vi "Teste Substrato Flexível 0.1_2025.vi"() -> ()   [LabVIEW 2019]
panel:
  in  "Zero":bool
  out "Posição":dbl
  out "T (s)":dbl format="%#_3g"
  out "F (hz)":dbl format="%#_3g"
  out "Tempo (s)":u32
  out "init":u32
  out "In LOOP":bool
  out "Close":bool
  out "Open":bool
  in  "Loop Stop":i32=50 min=1
  in  "Loop Stop":bool
  in  "stop":bool
  in  "Loop Infinito":bool
  out "Vel Cte":i32
  in  "Vel Loop":i32(slide)=20 min=10 max=200 step=5 scale=10.0..200.0
  in  "Jog":i32=10
  in  "Jog_s":string="10"
  in  "Desl_s":string="50"
  out "Contador":dbl format="%.2f"
  in  "Power Off":bool
  in  "Down":bool
  in  "Up":bool
  out "read buffer":string
  out "Direcção":bool
  out "error":errorcluster
  in  "Arduino":refnum<visa-resource-name>="COM3"
  # "Controle Mecanismo Teste de Substrato Flexível"
  # "LOEM"
  # "Velocidade de Deslocamento"
  # "Contador de Ciclos"
  # "Parar em ciclo"
  # "CONTROLE MANUAL"
  # "Pg Down"
  # "Pg Up"
  # "Steps"
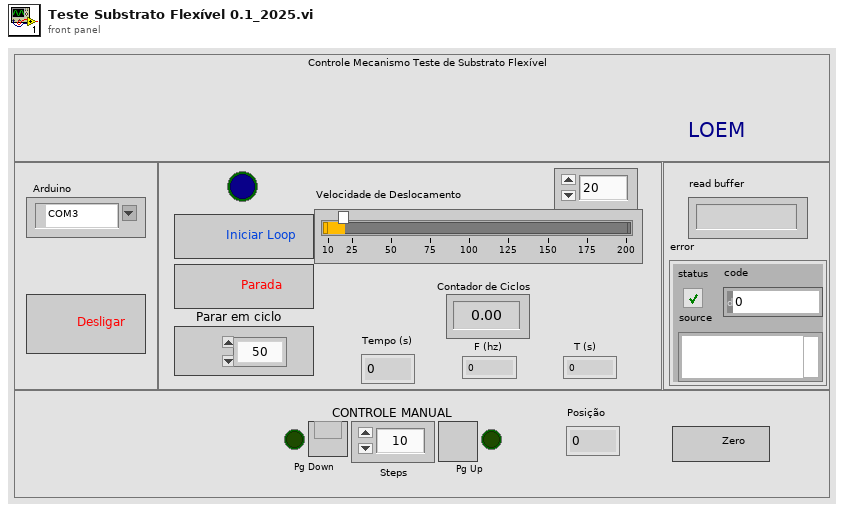
[diagram p1: front panel]
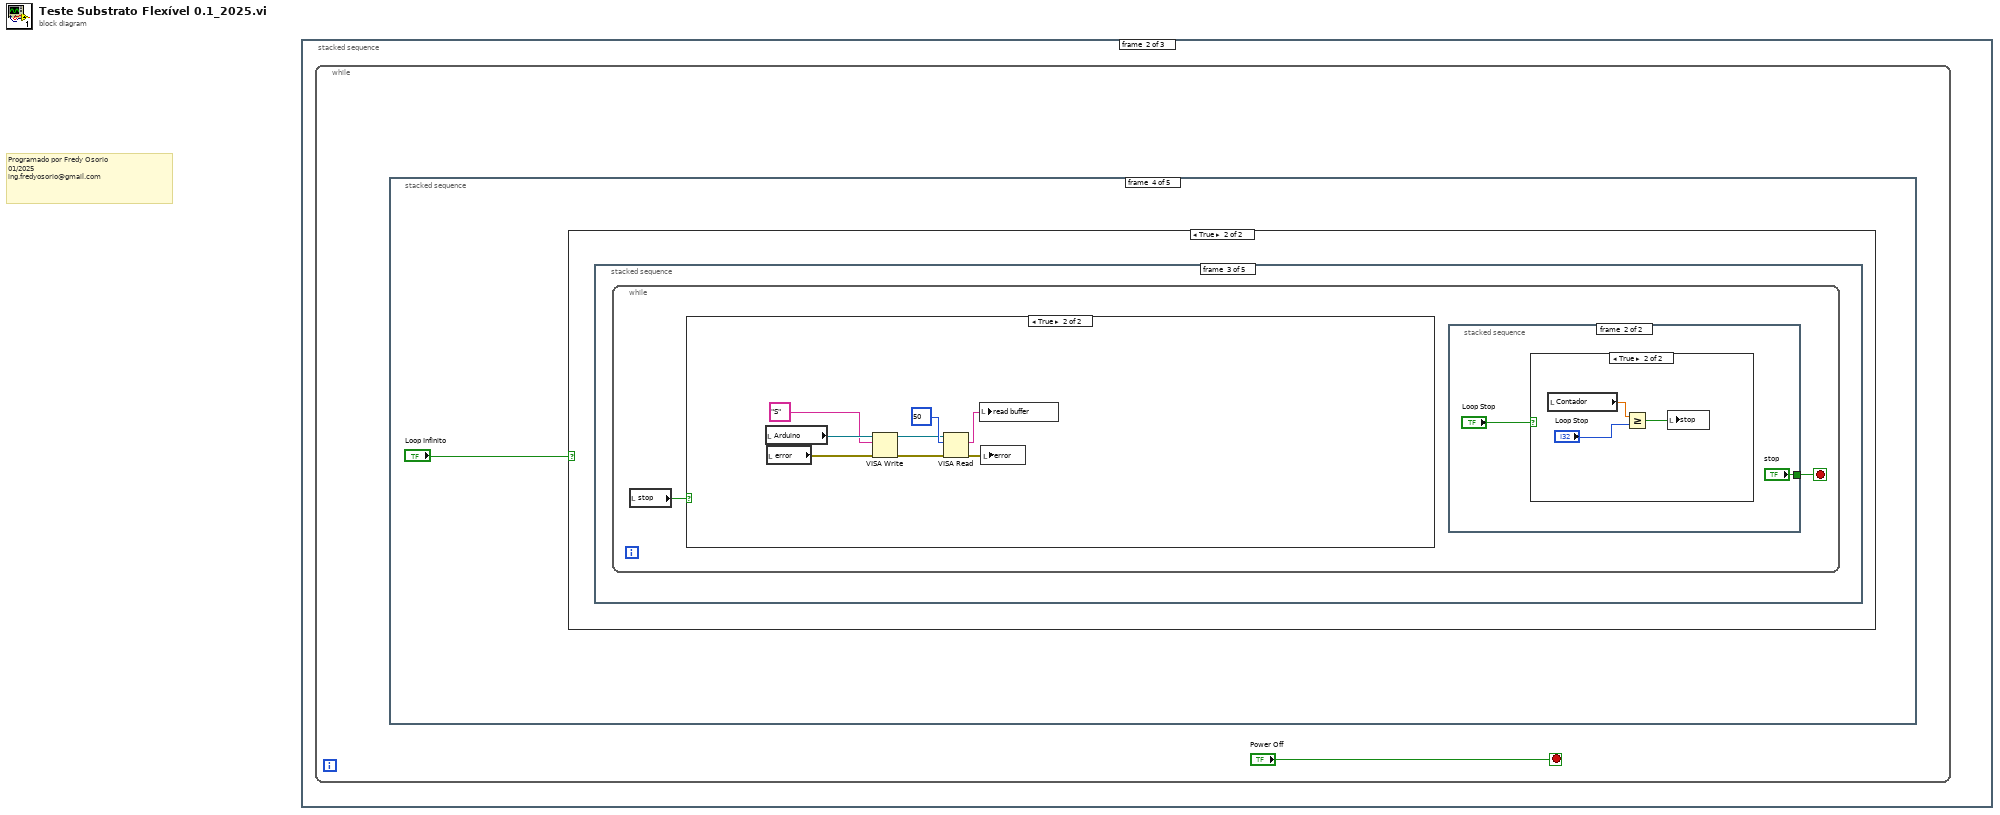
[diagram p0: block diagram]
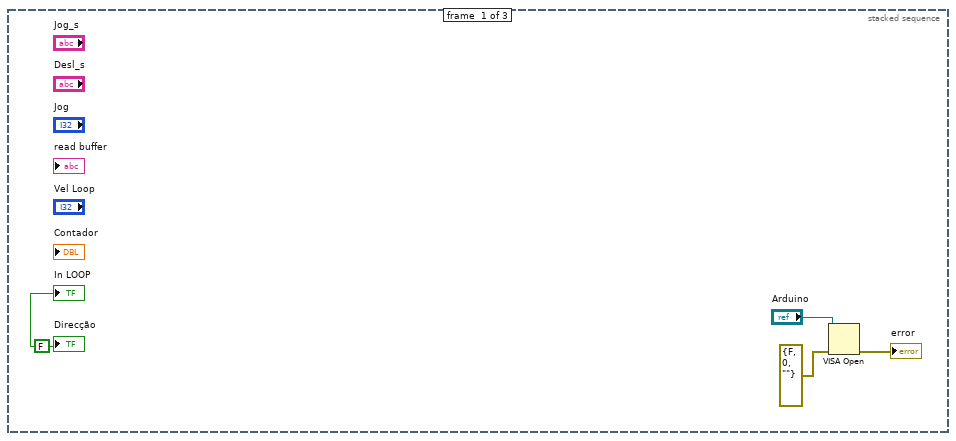
[diagram p2: hidden frame]
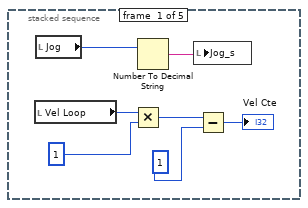
[diagram p3: hidden frame]
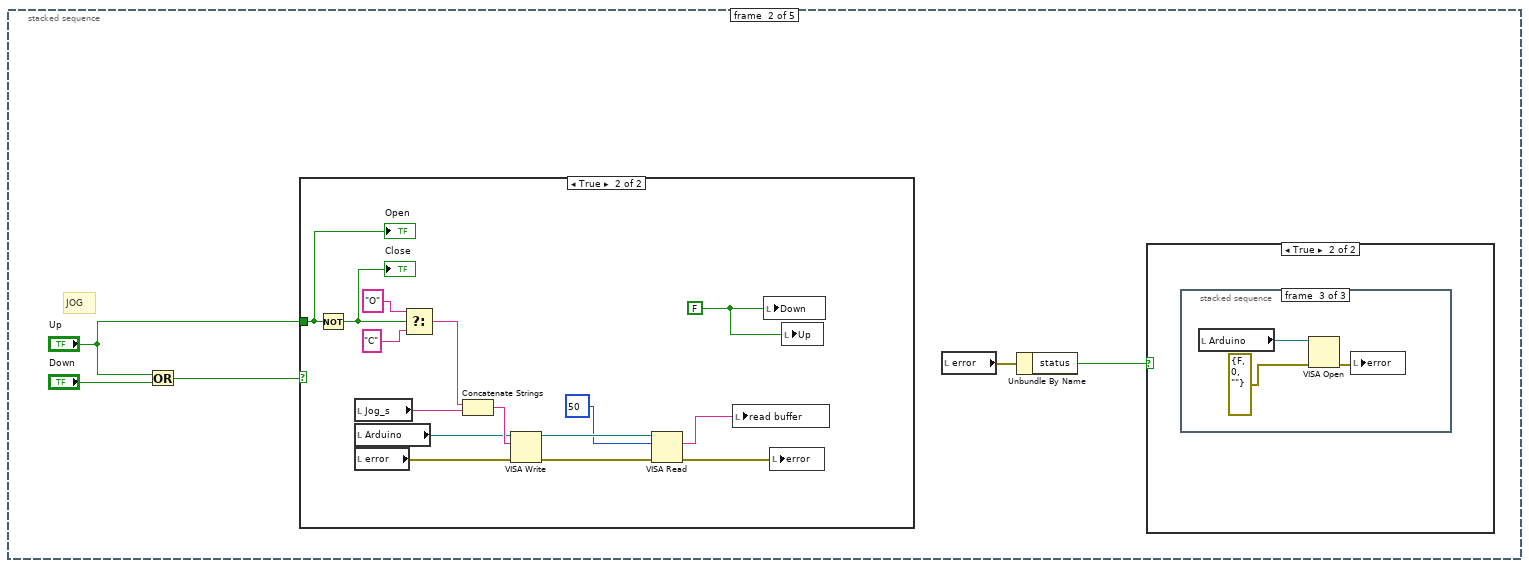
[diagram p4: hidden frame]
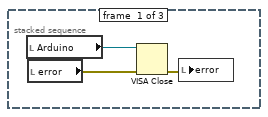
[diagram p6: hidden frame]
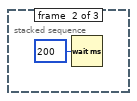
[diagram p7: hidden frame]
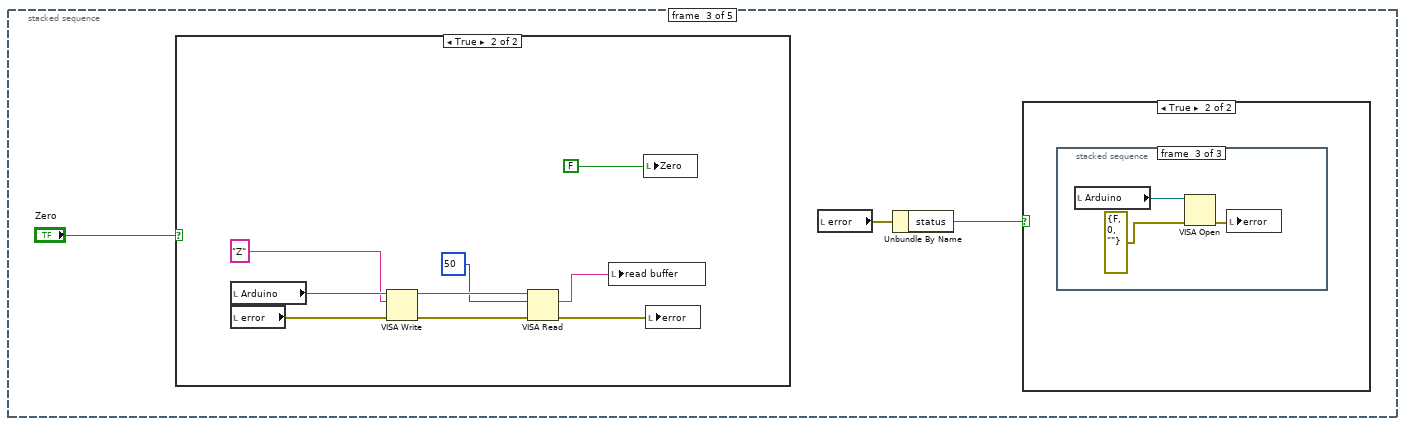
[diagram p9: hidden frame]
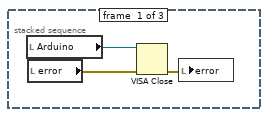
[diagram p11: hidden frame]
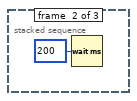
[diagram p12: hidden frame]
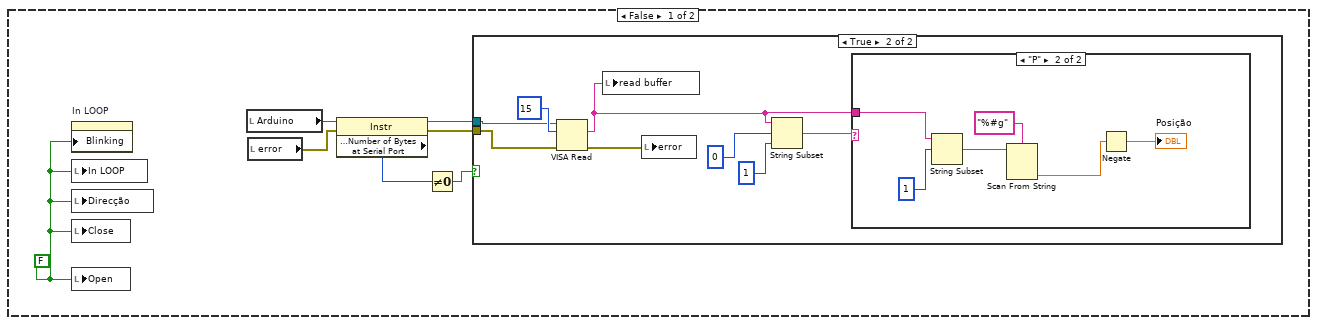
[diagram p14: hidden frame]
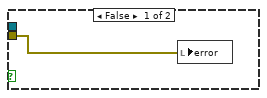
[diagram p15: hidden frame]
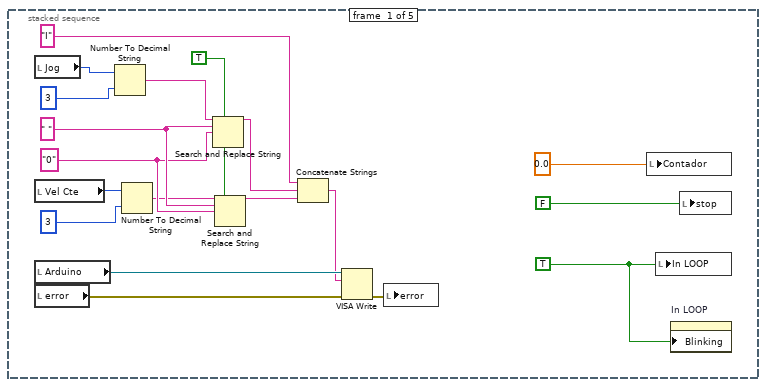
[diagram p17: hidden frame]
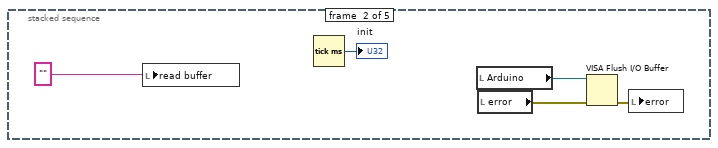
[diagram p18: hidden frame]
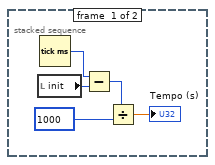
[diagram p19: hidden frame]
diagram:
  # "Programado por Fredy Osorio\n01/2025\ning.fredyosorio@gmail.com"
  n1 = stacked-sequence {
    frame #0 {
      w1 = FALSE ("In LOOP")
      n2 = VISA Open(error in (no error)=errorcluster {"status"=FALSE, "code"=0, "source"=""}, VISA resource name="Arduino") -> (error out=→"error":errorcluster)  [unwired: 3 in, 1 out]
      "Direcção" <- w1
      "In LOOP" <- w1
    }
    frame #1 {
      n3 = while {
        stop <- "Power Off" stop-if-true
        n4 = stacked-sequence {
          frame #0 {
            n5 = local read "Vel Loop"() -> (w9:i32)
            n6 = local read "Jog"() -> (w12:i32)
            n7 = Multiply(x=w9, y=1) -> (x*y=w10:i32)
            n8 = Number To Decimal String(number=w12) -> (decimal integer string=w11:string)  [unwired: 1 in]
            n9 = local write "Jog_s"(w11) -> ()
            n10 = Subtract(x=w10, y=1) -> (x-y=→"Vel Cte":i32)
          }
          frame #1 {
            # "JOG"
            n11 = Or(x="Up", y="Down") -> (x .or. y?=w16:bool)
            n12 = case shown="True" w16 {
              tunnel: "Up" -> [_ w29]
              frame False {
              }
              frame True {
                w31 = FALSE ("Previous")
                n13 = Not(x=w29) -> (.not. x?=w26:bool)
                "Close" <- w26
                n14 = local read "Jog_s"() -> (w30:string)
                n15 = local read "Arduino"() -> (w34:refnum<visa-resource-name>)
                n16 = local read "error"() -> (w35:errorcluster)
                n17 = Select(t="O", s=w26, f="C") -> (s? t:f=w25:string)
                n18 = Concatenate Strings(w25, w30) -> (w37:string)
                n19 = VISA Write(VISA resource name=w34, write buffer=w37, error in (no error)=w35) -> (VISA resource name out=w39:refnum<visa-resource-name>, error out=w38:errorcluster)  [unwired: 1 out]
                n20 = VISA Read(VISA resource name=w39, byte count=u32 50, error in (no error)=w38) -> (read buffer=w33:string, error out=w36:errorcluster)  [unwired: 2 out]
                n21 = local write "read buffer"(w33) -> ()
                n22 = local write "Down"(w31) -> ()
                n23 = local write "error"(w36) -> ()
                n24 = local write "Up"(w31) -> ()
                "Open" <- w29
              }
            }
            n25 = local read "error"() -> (w14:errorcluster)
            n26 = Unbundle By Name(w14) -> ("status"=w13:bool)
            n27 = case shown="True" w13 {
              frame False {
              }
              frame True {
                n28 = stacked-sequence {
                  frame #0 {
                    n29 = local read "Arduino"() -> (w18:refnum<visa-resource-name>)
                    n30 = local read "error"() -> (w19:errorcluster)
                    n31 = VISA Close(VISA resource name=w18, error in (no error)=w19) -> (error out=w20:errorcluster)
                    n32 = local write "error"(w20) -> ()
                  }
                  frame #1 {
                    n33 = Wait (ms)(milliseconds to wait=u32 200) -> ()  [unwired: 1 out]
                  }
                  frame #2 {
                    n34 = local read "Arduino"() -> (w23:refnum<visa-resource-name>)
                    n35 = VISA Open(error in (no error)=errorcluster {"status"=FALSE, "code"=0, "source"=""}, VISA resource name=w23) -> (error out=w24:errorcluster)  [unwired: 3 in, 1 out]
                    n36 = local write "error"(w24) -> ()
                  }
                }
              }
            }
          }
          frame #2 {
            n37 = case shown="True" "Zero" {
              frame False {
              }
              frame True {
                n38 = local read "Arduino"() -> (w54:refnum<visa-resource-name>)
                n39 = local read "error"() -> (w55:errorcluster)
                n40 = VISA Write(VISA resource name=w54, write buffer="Z", error in (no error)=w55) -> (VISA resource name out=w58:refnum<visa-resource-name>, error out=w57:errorcluster)  [unwired: 1 out]
                n41 = VISA Read(VISA resource name=w58, byte count=u32 50, error in (no error)=w57) -> (read buffer=w53:string, error out=w56:errorcluster)  [unwired: 2 out]
                n42 = local write "read buffer"(w53) -> ()
                n43 = local write "Zero"(FALSE ("Previous")) -> ()
                n44 = local write "error"(w56) -> ()
              }
            }
            n45 = local read "error"() -> (w42:errorcluster)
            n46 = Unbundle By Name(w42) -> ("status"=w41:bool)
            n47 = case shown="True" w41 {
              frame False {
              }
              frame True {
                n48 = stacked-sequence {
                  frame #0 {
                    n49 = local read "Arduino"() -> (w43:refnum<visa-resource-name>)
                    n50 = local read "error"() -> (w44:errorcluster)
                    n51 = VISA Close(VISA resource name=w43, error in (no error)=w44) -> (error out=w45:errorcluster)
                    n52 = local write "error"(w45) -> ()
                  }
                  frame #1 {
                    n53 = Wait (ms)(milliseconds to wait=u32 200) -> ()  [unwired: 1 out]
                  }
                  frame #2 {
                    n54 = local read "Arduino"() -> (w48:refnum<visa-resource-name>)
                    n55 = VISA Open(error in (no error)=errorcluster {"status"=FALSE, "code"=0, "source"=""}, VISA resource name=w48) -> (error out=w49:errorcluster)  [unwired: 3 in, 1 out]
                    n56 = local write "error"(w49) -> ()
                  }
                }
              }
            }
          }
          frame #3 {
            n57 = case shown="True" "Loop Infinito" {
              frame False {
                w60 = FALSE ("Open")
                n58 = property on="In LOOP" class="Bool (strict)"("Blinking"=w60) -> ()  [unwired: 2 in, 2 out]
                n59 = local write "In LOOP"(w60) -> ()
                n60 = local write "Direcção"(w60) -> ()
                n61 = local write "Close"(w60) -> ()
                n62 = local write "Open"(w60) -> ()
                n63 = local read "Arduino"() -> (w61:refnum<visa-resource-name>)
                n64 = local read "error"() -> (w63:errorcluster)
                n65 = property class="Instr"(reference=w61, error in=w63) -> (reference out=w62:refnum<visa-resource-name>, error out=w64:errorcluster, "Serial Settings:Number of Bytes at Serial Port"=w66:u32)
                n66 = Not Equal To 0?(x=w66) -> (x != 0?=w65:bool)
                n67 = case shown="True" w65 {
                  tunnel: w62 -> [_ w73]
                  tunnel: w64 -> [w67 w72]
                  frame False {
                    n68 = local write "error"(w67) -> ()
                  }
                  frame True {
                    n69 = VISA Read(VISA resource name=w73, byte count=u32 15, error in (no error)=w72) -> (read buffer=w69:string, error out=w75:errorcluster)  [unwired: 2 out]
                    n70 = local write "read buffer"(w69) -> ()
                    n71 = local write "error"(w75) -> ()
                    n72 = String Subset(string=w69, offset (0)=0, length (rest)=1 ("length (rest)")) -> (substring=w68:string)
                    n73 = case shown="\"P\"" w68 {
                      tunnel: w69 -> [_ w80]
                      frame "False", Default {
                      }
                      frame "P" {
                        n74 = String Subset(string=w80, offset (0)=1 ("length (rest)")) -> (substring=w77:string)  [unwired: 1 in]
                        n75 = Scan From String(format string="%#g", input string=w77) -> (output 1=w79:dbl)  [unwired: 3 in, 3 out]
                        n76 = Negate(x=w79) -> (-x=→"Posição":dbl)
                      }
                    }
                  }
                }
              }
              frame True {
                n77 = stacked-sequence {
                  frame #0 {
                    w82 = TRUE ("replace all? (F)")
                    w87 = "0" ("replace string (\"\")")
                    w88 = " " ("search string")
                    w92 = TRUE ("In LOOP")
                    n78 = local read "Jog"() -> (w93:i32)
                    n79 = local read "Vel Cte"() -> (w86:i32)
                    n80 = local read "Arduino"() -> (w98:refnum<visa-resource-name>)
                    n81 = local read "error"() -> (w99:errorcluster)
                    n82 = Number To Decimal String(number=w93, width (-)=i16 3) -> (decimal integer string=w91:string)
                    n83 = Number To Decimal String(number=w86, width (-)=i16 3) -> (decimal integer string=w85:string)
                    n84 = Search and Replace String(replace all?=w82, input string=w91, search string=w88, replace string=w87) -> (result string=w90:string)  [unwired: 4 in, 3 out]
                    n85 = Search and Replace String(replace all?=w82, input string=w85, search string=w88, replace string=w87) -> (result string=w89:string)  [unwired: 4 in, 3 out]
                    n86 = Concatenate Strings("I" ("write buffer"), w90, w89) -> (w97:string)
                    n87 = VISA Write(VISA resource name=w98, write buffer=w97, error in (no error)=w99) -> (error out=w100:errorcluster)  [unwired: 2 out]
                    n88 = local write "error"(w100) -> ()
                    n89 = local write "Contador"(0.0 ("Contador")) -> ()
                    n90 = local write "In LOOP"(w92) -> ()
                    n91 = property on="In LOOP" class="Bool (strict)"("Blinking"=w92) -> ()  [unwired: 2 in, 2 out]
                    n92 = local write "stop"(FALSE ("stop")) -> ()
                  }
                  frame #1 {
                    n93 = local write "read buffer"("" ("read buffer")) -> ()
                    n94 = Tick Count (ms)() -> (millisecond timer value=→"init":u32)
                    n95 = local read "Arduino"() -> (w103:refnum<visa-resource-name>)
                    n96 = local read "error"() -> (w104:errorcluster)
                    n97 = VISA Flush I/O Buffer(VISA resource name=w103, error in (no error)=w104) -> (error out=w105:errorcluster)  [unwired: 1 in, 1 out]
                    n98 = local write "error"(w105) -> ()
                  }
                  frame #2 {
                    n99 = while {
                      stop <- w107 stop-if-true
                      n100 = local read "stop"() -> (w106:bool)
                      n101 = case shown="True" w106 {
                        frame False {
                          n102 = local read "Arduino"() -> (w118:refnum<visa-resource-name>)
                          n103 = local read "error"() -> (w120:errorcluster)
                          n104 = property class="Instr"(reference=w118, error in=w120) -> (reference out=w119:refnum<visa-resource-name>, error out=w121:errorcluster, "Serial Settings:Number of Bytes at Serial Port"=w123:u32)
                          n105 = Not Equal To 0?(x=w123) -> (x != 0?=w122:bool)
                          n106 = case shown="True" w122 {
                            tunnel: w119 -> [_ w126]
                            tunnel: w121 -> [w124 w125]
                            frame False {
                              n107 = local write "error"(w124) -> ()
                            }
                            frame True {
                              n108 = stacked-sequence {
                                tunnel: w126 -> [w130 _ _ _]
                                tunnel: w125 -> [w128 _ _ _]
                                frame #0 {
                                n109 = VISA Read(VISA resource name=w130, byte count=u32 15, error in (no error)=w128) -> (read buffer=w127:string, error out=w131:errorcluster)  [unwired: 2 out]
                                n110 = local write "read buffer"(w127) -> ()
                                n111 = local write "error"(w131) -> ()
                                }
                                frame #1 {
                                n112 = local read "read buffer"() -> (w135:string)
                                n113 = Search and Replace String(input string=w135, search string=".", replace string="," ("replace string (\"\")")) -> (result string=w134:string)  [unwired: 5 in, 3 out]
                                n114 = local write "read buffer"(w134) -> ()
                                }
                                frame #2 {
                                n115 = local read "read buffer"() -> (w136:string)
                                n116 = String Subset(string=w136, offset (0)=0, length (rest)=1 ("length (rest)")) -> (substring=w137:string)
                                n117 = case shown="\"L\"" w137 {
                                tunnel: w136 -> [_ w143]
                                frame "False", Default {
                                }
                                frame "L" {
                                n118 = Search and Replace String(input string=w143, search string=",", replace string="." ("replace string (\"\")")) -> (result string=w142:string)  [unwired: 5 in, 3 out]
                                n119 = String Subset(string=w142, offset (0)=1) -> (substring=w145:string)  [unwired: 1 in]
                                n120 = Scan From String(format string="%#g", input string=w145) -> (output 1=w146:dbl)  [unwired: 3 in, 3 out]
                                n121 = local write "Contador"(w146) -> ()
                                }
                                }
                                }
                                frame #3 {
                                n122 = local read "Tempo (s)"() -> (w149:u32)
                                n123 = local read "Contador"() -> (w150:dbl)
                                n124 = Divide(x=w150, y=w149) -> (x/y=→"F (hz)":dbl)
                                n125 = Divide(x=w149, y=w150) -> (x/y=→"T (s)":dbl)
                                }
                              }
                            }
                          }
                        }
                        frame True {
                          n126 = local read "Arduino"() -> (w159:refnum<visa-resource-name>)
                          n127 = local read "error"() -> (w158:errorcluster)
                          n128 = VISA Write(VISA resource name=w159, write buffer="S", error in (no error)=w158) -> (VISA resource name out=w154:refnum<visa-resource-name>, error out=w156:errorcluster)  [unwired: 1 out]
                          n129 = VISA Read(VISA resource name=w154, byte count=u32 50, error in (no error)=w156) -> (read buffer=w152:string, error out=w157:errorcluster)  [unwired: 2 out]
                          n130 = local write "read buffer"(w152) -> ()
                          n131 = local write "error"(w157) -> ()
                        }
                      }
                      n132 = stacked-sequence {
                        tunnel: [_ "stop"] -> w107
                        frame #0 {
                          n133 = local read "init"() -> (w112:u32)
                          n134 = Tick Count (ms)() -> (millisecond timer value=w111:u32)
                          n135 = Subtract(x=w111, y=w112) -> (x-y=w110:u32)
                          n136 = Divide(x=w110, y=u32 1000) -> (x/y=→"Tempo (s)":dbl)
                        }
                        frame #1 {
                          n137 = case shown="True" "Loop Stop" {
                            frame False {
                            }
                            frame True {
                              n138 = local read "Contador"() -> (w117:dbl)
                              n139 = Greater Or Equal?(x=w117, y="Loop Stop") -> (x >= y?=w115:bool)
                              n140 = local write "stop"(w115) -> ()
                            }
                          }
                        }
                      }
                    }
                  }
                  frame #3 {
                    n141 = local read "Arduino"() -> (w164:refnum<visa-resource-name>)
                    n142 = local read "error"() -> (w165:errorcluster)
                    n143 = VISA Write(VISA resource name=w164, write buffer="S", error in (no error)=w165) -> (VISA resource name out=w168:refnum<visa-resource-name>, error out=w167:errorcluster)  [unwired: 1 out]
                    n144 = VISA Read(VISA resource name=w168, byte count=u32 50, error in (no error)=w167) -> (read buffer=w163:string, error out=w166:errorcluster)  [unwired: 2 out]
                    n145 = local write "read buffer"(w163) -> ()
                    n146 = local write "error"(w166) -> ()
                    n147 = local write "stop"(FALSE ("stop")) -> ()
                  }
                  frame #4 {
                    n148 = Wait (ms)(milliseconds to wait=u32 500) -> ()  [unwired: 1 out]
                  }
                }
              }
            }
          }
          frame #4 {
            n149 = local read "stop"() -> (w170:bool)
            n150 = case shown="True" w170 {
              frame False {
              }
              frame True {
                n151 = local read "Arduino"() -> (w173:refnum<visa-resource-name>)
                n152 = local read "error"() -> (w174:errorcluster)
                n153 = VISA Write(VISA resource name=w173, write buffer="S", error in (no error)=w174) -> (VISA resource name out=w178:refnum<visa-resource-name>, error out=w176:errorcluster)  [unwired: 1 out]
                n154 = VISA Read(VISA resource name=w178, byte count=u32 50, error in (no error)=w176) -> (read buffer=w180:string, error out=w175:errorcluster)  [unwired: 2 out]
                n155 = local write "read buffer"(w180) -> ()
                n156 = local write "error"(w175) -> ()
                n157 = local write "stop"(FALSE ("stop")) -> ()
              }
            }
            n158 = Wait (ms)(milliseconds to wait=u32 150) -> ()  [unwired: 1 out]
          }
        }
      }
    }
    frame #2 {
      n159 = local read "Arduino"() -> (w183:refnum<visa-resource-name>)
      n160 = local read "error"() -> (w182:errorcluster)
      n161 = VISA Close(VISA resource name=w183, error in (no error)=w182) -> (error out=w181:errorcluster)
      n162 = local write "error"(w181) -> ()
    }
  }
